vi "LimitFlagActionSoftLinearizedZ.vi"(4 "Soft":bool, 5 "Axis limit flag":bool, 6 "Old Control":dbl, 7 "Global limit flag active":dbl, 8 "Stop motors global":bool, 9 "Stop motor local":bool, 10 "Axis control signal":dbl) -> (0 "Slider control":dbl, 1 "PWM Brake":u32, 2 "PWM Direction":u32, 3 "PWM width":u32)   [LabVIEW 2009]
uses:
  <vilib>/imath/engines/lvmath2/RunTimeEngine/ErrorHandling/NIMS_Finalize Error.vi
  <vilib>/imath/engines/lvmath2/RunTimeEngine/Parser/MC_Version.vi
  <vilib>/imath/engines/lvmath2/RunTimeEngine/NodeEndStatement/NIMS_NodeEndStatement_Output.vi
  <instcachedir>/0/NIMS_NodeEndStatement_Output_53EC0D466D134D7ABD903AC30B43404B.lvgen/NIMS_NodeEndStatement_Output_53EC0D466D134D7ABD903AC30B43404B_002.vi
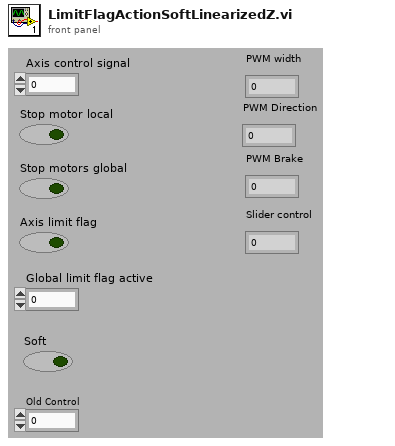
[diagram p1: front panel]
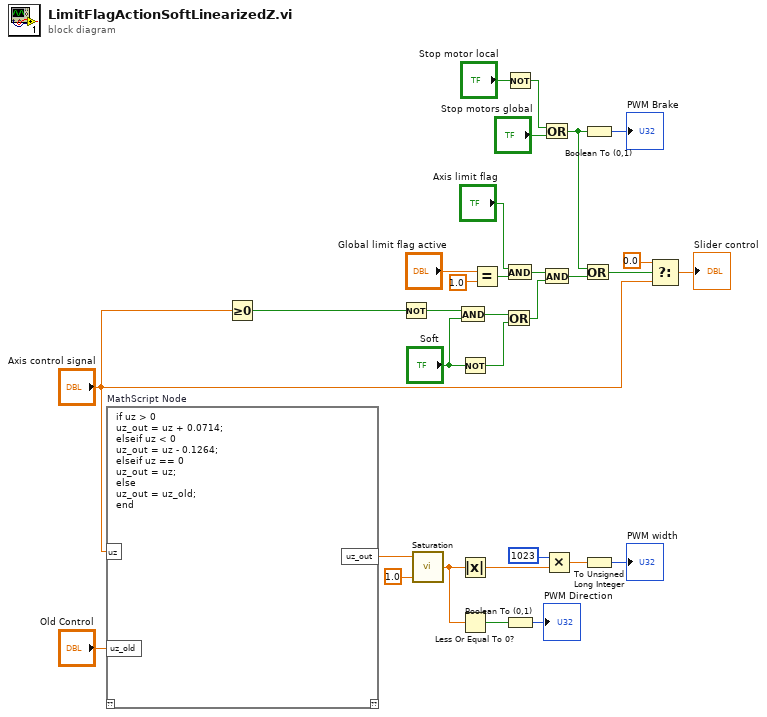
[diagram p0: block diagram]
diagram:
  n1 = mathscript code="if uz > 0\nuz_out = uz + 0.0714;\nelseif uz < 0\nuz_out = uz - 0.1264;\nelseif uz == 0\nuz_out = uz;\nelse\nuz_out = uz_old;\nend"("uz"="Axis control signal", "uz_old"="Old Control") -> ("uz_out"=w3:dbl)  [unwired: 1 in, 1 out]
  n2 = Greater Or Equal To 0?(x="Axis control signal") -> (x >= 0?=w11:bool)
  n3 = Not(x=w11) -> (.not. x?=w10:bool)
  n4 = call "Saturation.vi"("Limit"=1.0, "Input"=w3) -> ("Output"=w1:dbl)
  n5 = And(x=w10, y="Soft") -> (x .and. y?=w9:bool)
  n6 = Not(x="Soft") -> (.not. x?=w8:bool)
  n7 = Absolute Value(x=w1) -> (abs(x)=w22:dbl)
  n8 = Less Or Equal To 0?(x=w1) -> (x <= 0?=w19:bool)
  n9 = Equal?(x="Global limit flag active", y=1.0) -> (x = y?=w29:bool)
  n10 = Or(x=w9, y=w8) -> (x .or. y?=w6:bool)
  n11 = Not(x="Stop motor local") -> (.not. x?=w31:bool)
  n12 = And(x="Axis limit flag", y=w29) -> (x .and. y?=w12:bool)
  n13 = Boolean To (0,1)(Boolean=w19) -> (0, 1=→"PWM Direction":i16)
  n14 = Or(x=w31, y="Stop motors global") -> (x .or. y?=w15:bool)
  n15 = And(x=w12, y=w6) -> (x .and. y?=w13:bool)
  n16 = Multiply(x=1023, y=w22) -> (x*y=w20:dbl)
  n17 = Or(x=w15, y=w13) -> (x .or. y?=w16:bool)
  n18 = Boolean To (0,1)(Boolean=w15) -> (0, 1=→"PWM Brake":i16)
  n19 = To Unsigned Long Integer(number=w20) -> (unsigned 32bit integer=→"PWM width":u32)
  n20 = Select(t=0.0, s=w16, f="Axis control signal") -> (s? t:f=→"Slider control":dbl)
